vi "FPGA ParseCompass.vi"(10 "Serial Byte":u8) -> (2 "Heading":T1)   [LabVIEW 2009]
panel:
  in  "Heading Init":T1 {"Yaw" format="%.42g"; "Pitch" format="%.42g"; "Roll" format="%.42g"}
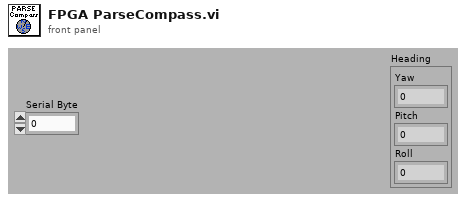
[diagram p1: front panel]
types:
  T1 = cluster{"Yaw":fxp<+/-,64,32>, "Pitch":fxp<+/-,64,32>, "Roll":fxp<+/-,64,32>}
  T2 = enum16{"Initialize", "Yaw", "Pitch", "Roll", "Done"}
  T3 = enum16{"Wait for $", "Check VNYPR", "skip ,", "read +-", "read numbers"}
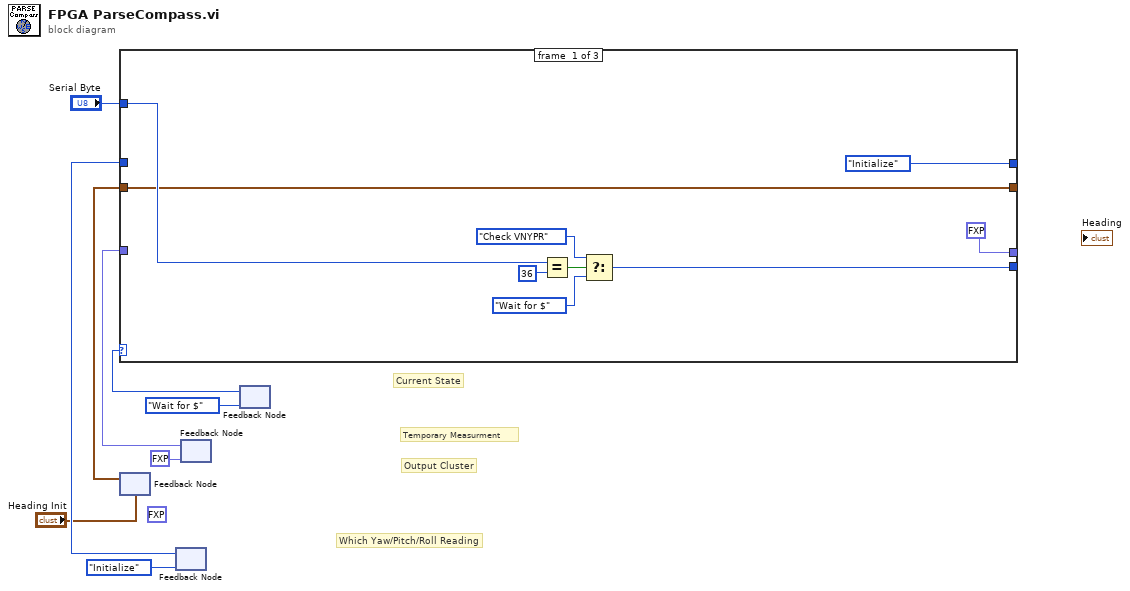
[diagram p0: block diagram]
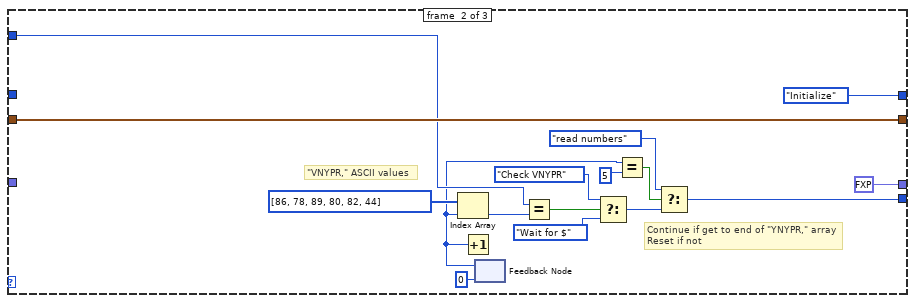
[diagram p2: hidden frame]
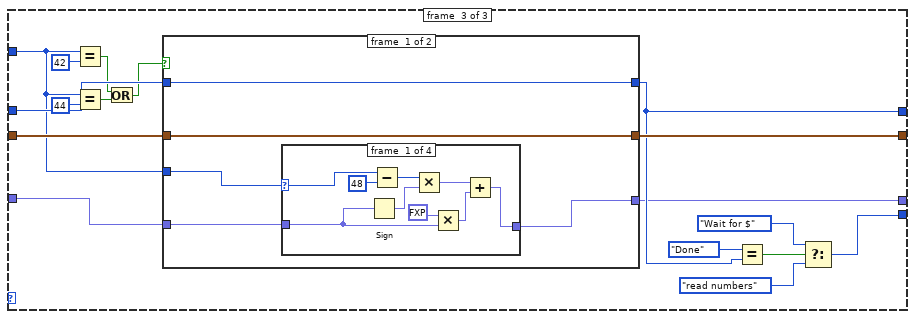
[diagram p3: hidden frame]
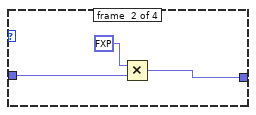
[diagram p4: hidden frame]
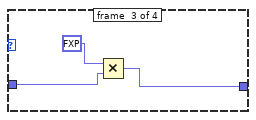
[diagram p5: hidden frame]
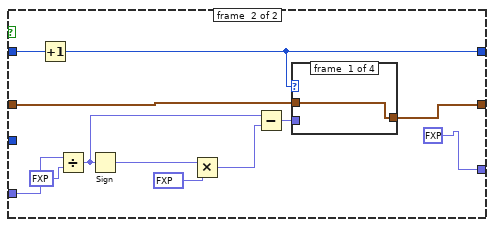
[diagram p7: hidden frame]
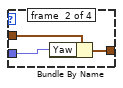
[diagram p8: hidden frame]
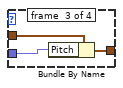
[diagram p9: hidden frame]
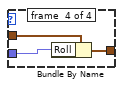
[diagram p10: hidden frame]
diagram:
  (unwired) fxp<+/-,32,12> 0.0 ("Yaw")
  # "Output Cluster"
  # "Temporary Measurment"
  # "Current State"
  # "Which Yaw/Pitch/Roll Reading"
  n1 = feedback #1("Heading Init") -> (w6:T1)
  n2 = feedback #2(T2."Initialize" ("f")) -> (w3:T2)
  n3 = feedback #3(fxp<+/-,64,32> 1.0 ("Yaw")) -> (w9:fxp<+/-,64,2047>)
  n4 = feedback #4(T3."Wait for $" ("f")) -> (w10:T3)
  n5 = case shown="\"Check VNYPR\"" w10 {
    tunnel: [w17 w25 w42] -> w13
    tunnel: "Serial Byte" -> [w22 w31 w40]
    tunnel: w9 -> [_ _ w43]
    tunnel: [fxp<+/-,32,12> 1.0 ("Yaw") fxp<+/-,32,12> 1.0 ("Yaw") w44] -> w2
    tunnel: [w16 w32 w54] -> w7
    tunnel: w6 -> [w16 w32 w55]
    tunnel: [T2."Initialize" ("f") T2."Initialize" ("f") w52] -> w4
    tunnel: w3 -> [_ _ w53]
    frame #0 {
      n6 = Equal?(x=w22, y=u8 36) -> (x = y?=w20:bool)
      n7 = Select(t=T3."Check VNYPR" ("f"), s=w20, f=T3."Wait for $") -> (s? t:f=w17:T3)
    }
    frame #1 {
      # "\"VNYPR,\" ASCII values"
      # "Continue if get to end of \"YNYPR,\" array\nReset if not"
      n8 = feedback #5(u8 0 ("Serial Byte")) -> (w24:u8)
      n9 = Index Array(array=u8[] [86, 78, 89, 80, 82, 44], index=w24) -> (element=w37:u8)
      n10 = Increment(x=w24) -> (x+1=w33:u8)
      n11 = Equal?(x=w31, y=w37) -> (x = y?=w34:bool)
      n12 = Select(t=T3."Check VNYPR" ("f"), s=w34, f=T3."Wait for $") -> (s? t:f=w29:T3)
      n13 = Equal?(x=w24, y=u8 5) -> (x = y?=w28:bool)
      n14 = Select(t=T3."read numbers", s=w28, f=w29) -> (s? t:f=w25:T3)
    }
    frame #2 {
      n15 = Equal?(x=w40, y=u8 42) -> (x = y?=w46:bool)
      n16 = Equal?(x=w40, y=u8 44) -> (x = y?=w47:bool)
      n17 = Or(x=w46, y=w47) -> (x .or. y?=w45:bool)
      n18 = case shown="True" w45 {
        tunnel: w55 -> [w61 w89]
        tunnel: [w61 w88] -> w54
        tunnel: [w60 w86] -> w52
        tunnel: w53 -> [w60 w87]
        tunnel: [w57 fxp<+/-,32,12> 1.0 ("Yaw")] -> w44
        tunnel: w43 -> [w58 w85]
        tunnel: w40 -> [w59 _]
        frame #0 {
          n19 = case shown="46" w59 {
            selector: w59 -> [w68 _ _ _]
            tunnel: w58 -> [w69 w73 w76 w77]
            tunnel: [w63 w72 w75 w77] -> w57
            frame #0 {
              n20 = Sign(1:w69) -> (0:w65:fxp<+/-,2,2>)
              n21 = Subtract(x=w68, y=u8 48) -> (x-y=w66:u8)
              n22 = Multiply(x=w66, y=w65) -> (x*y=w64:fxp<+/-,9,9>)
              n23 = Multiply(x=fxp<+/-,32,12> 10.0 ("Yaw"), y=w69) -> (x*y=w70:fxp)
              n24 = Add(x=w64, y=w70) -> (x+y=w63:fxp)
            }
            frame #1 {
              n25 = Multiply(x=fxp<+/-,32,12> 1.0 ("Yaw"), y=w73) -> (x*y=w72:fxp)
            }
            frame #2 {
              n26 = Multiply(x=fxp<+/-,32,12> -1.0 ("Yaw"), y=w76) -> (x*y=w75:fxp)
            }
            frame #3 {
            }
          }
        }
        frame #1 {
          n27 = Increment(x=w87) -> (x+1=w86:T2)
          n28 = Divide(x=w85, y=fxp<+/-,32,12> 100.0 ("Yaw")) -> (x/y=w83:fxp)
          n29 = Sign(1:w83) -> (0:w81:fxp<+/-,2,2>)
          n30 = Multiply(x=w81, y=fxp<+/-,32,12> 1000.0 ("Yaw")) -> (x*y=w82:fxp<+/-,33,13>)
          n31 = Subtract(x=w83, y=w82) -> (x-y=w84:fxp)
          n32 = case shown="\"Pitch\"" w86 {
            tunnel: [w90 w93 w96 w99] -> w88
            tunnel: w89 -> [w90 w92 w95 w98]
            tunnel: w84 -> [_ w91 w94 w97]
            frame #0 {
            }
            frame #1 {
              n33 = Bundle By Name(cluster=w92, "Yaw"=w91) -> (w93:T1)
            }
            frame #2 {
              n34 = Bundle By Name(cluster=w95, "Pitch"=w94) -> (w96:T1)
            }
            frame #3 {
              n35 = Bundle By Name(cluster=w98, "Roll"=w97) -> (w99:T1)
            }
          }
        }
      }
      n36 = Equal?(x=T2."Done", y=w52) -> (x = y?=w50:bool)
      n37 = Select(t=T3."Wait for $" ("f"), s=w50, f=T3."read numbers") -> (s? t:f=w42:T3)
    }
  }
